vi "getAllAttributes.vi"(8 "error in (no error)":errorcluster, 11 "camera in":refnum<class "camera.lvclass">) -> (0 "error out":errorcluster, 2 "Attribute Information Array":T2(array[cluster]), 3 "camera out":refnum<class "camera.lvclass">)   [LabVIEW 2017, in "camera.lvclass"]
uses:
  camera.lvclass
  <vilib>/vision/driver/IMAQdx.llb/IMAQdx Attribute Type.ctl
  <vilib>/vision/driver/NI_Vision_Acquisition_Software.lvlib
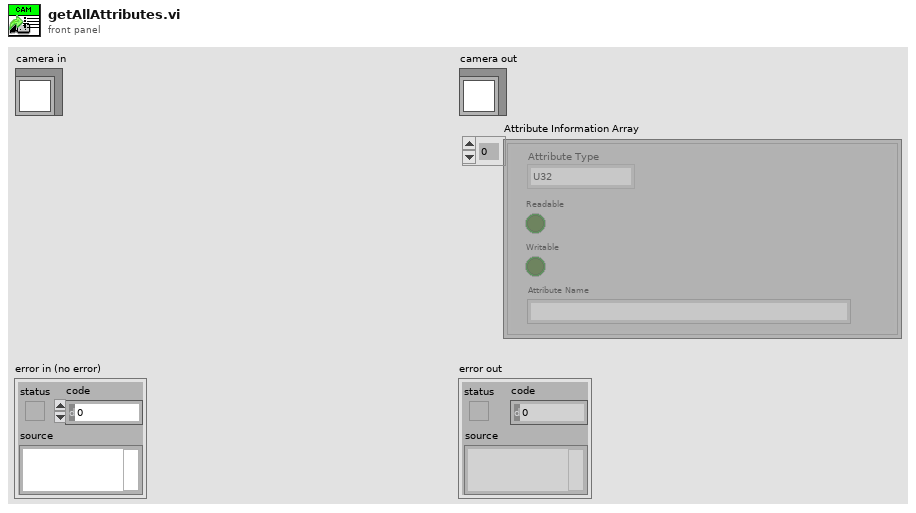
[diagram p1: front panel]
types:
  T1 = typedef "NI_Vision_Acquisition_Software.lvlib/IMAQdx Attribute Type.ctl" = enum32{"U32", "I64", "DBL", "String", "Enum", "Bool", "Command"}
  T2 = cluster{"Attribute Type":T1, "Readable":bool, "Writable":bool, "Attribute Name":string}[]
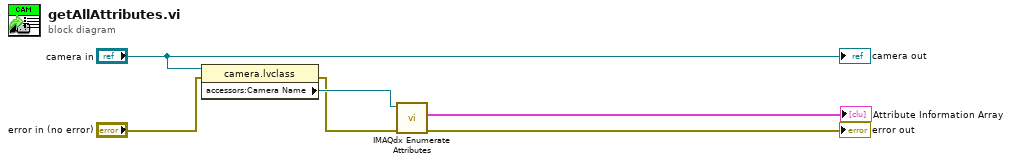
[diagram p0: block diagram]
diagram:
  n1 = property class="camera.lvclass"(reference="camera in", error in="error in (no error)") -> (error out=w3:errorcluster, "accessors:Camera Name"=w5:refnum<k21>)  [unwired: 1 out]
  n2 = call <vilib>:"IMAQdx Enumerate Attributes.vi"("error in"=w3, "Session In"=w5) -> ("error out"=→"error out":errorcluster, "Attribute Information Array"=→"Attribute Information Array":T2)  [unwired: 7 in, 1 out]
  "camera out" <- "camera in"
